vi "Demo_Ita.vi"() -> ()   [LabVIEW 2019]
uses:
  ByteQXAPIBase/ByteQXAPIBase.lvclass
  ByteQXAPIBase/FetchCalibration/Converted_Slug_Cluster.ctl
  ByteQXAPIBase/CalibrationMeasurements/CalibMeasure.ctl
  6d3d0a70-a223-4ddd-b0d3-7207305fe689.vi
  85eea304-0067-4311-882a-d02f57de18c2.vi
panel:
  out "Valore misurato":string
  out "Valore di riferimento":string
  in  "Start":bool
  in  "Send":bool
  out "Infobox":string
  out "Strumenti da calibrare":i32(listbox)
  in  "Exit":bool=TRUE
  in  "Calibrate":bool
  in  "error out":errorcluster
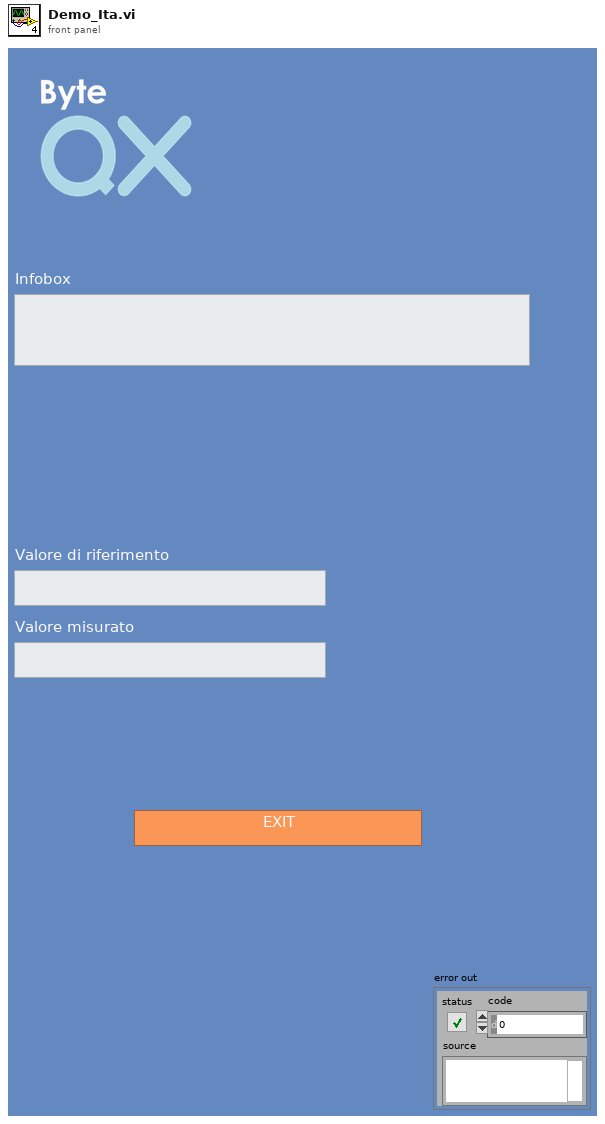
[diagram p1: front panel]
types:
  T1 = cluster{"nome":string, cluster{"Measurement_Id":i32, "Passed?":bool}[]}[]
  T2 = typedef "ByteQXWebAPI.lvlib/ByteQXAPIBase.lvclass/CalibMeasure.ctl" = cluster{"controls":cluster{"id":u16, "descrizione":string, "numero_misure_necessarie":u16, "riferimento_obiettivo":dbl, "mpe_max":dbl, "mpe_min":dbl, "deviazione_standard":dbl, "incertezza":dbl, "numero_misure_effettuate":u32, "temperatura_c":dbl, "umidita":dbl, "strumento_riferimento":cluster{"id":u16, "nome":string}[]}[]}
  T3 = typedef "ByteQXWebAPI.lvlib/ByteQXAPIBase.lvclass/Converted_Slug_Cluster.ctl" = cluster{"id":u32, "instrument":string, "name":string, "date":timestamp}
  T4 = cluster{"ByteQXAPIBase in":refnum<class "ByteQXAPIBase.lvclass">, "Expired_Instruments":T3[], "Calibrations":T2, "Strumenti_calibrati":cluster{"nome":string, cluster{"Measurement_Id":i32, "Passed?":bool}[]}[], "Instr_index":i32, "Calib_index":i32, "Instruments_Slug":string[], "ID_failed":u32, "Measure_Index":u32}
  T5 = cluster{"id":u16, "descrizione":string, "numero_misure_necessarie":u16, "riferimento_obiettivo":dbl, "mpe_max":dbl, "mpe_min":dbl, "deviazione_standard":dbl, "incertezza":dbl, "numero_misure_effettuate":u32, "temperatura_c":dbl, "umidita":dbl, "strumento_riferimento":cluster{"id":u16, "nome":string}[]}[]
  T6 = cluster{"id":u16, "descrizione":string, "numero_misure_necessarie":u16, "riferimento_obiettivo":dbl, "mpe_max":dbl, "mpe_min":dbl, "deviazione_standard":dbl, "incertezza":dbl, "numero_misure_effettuate":u32, "temperatura_c":dbl, "umidita":dbl, "strumento_riferimento":cluster{"id":u16, "nome":string}[]}
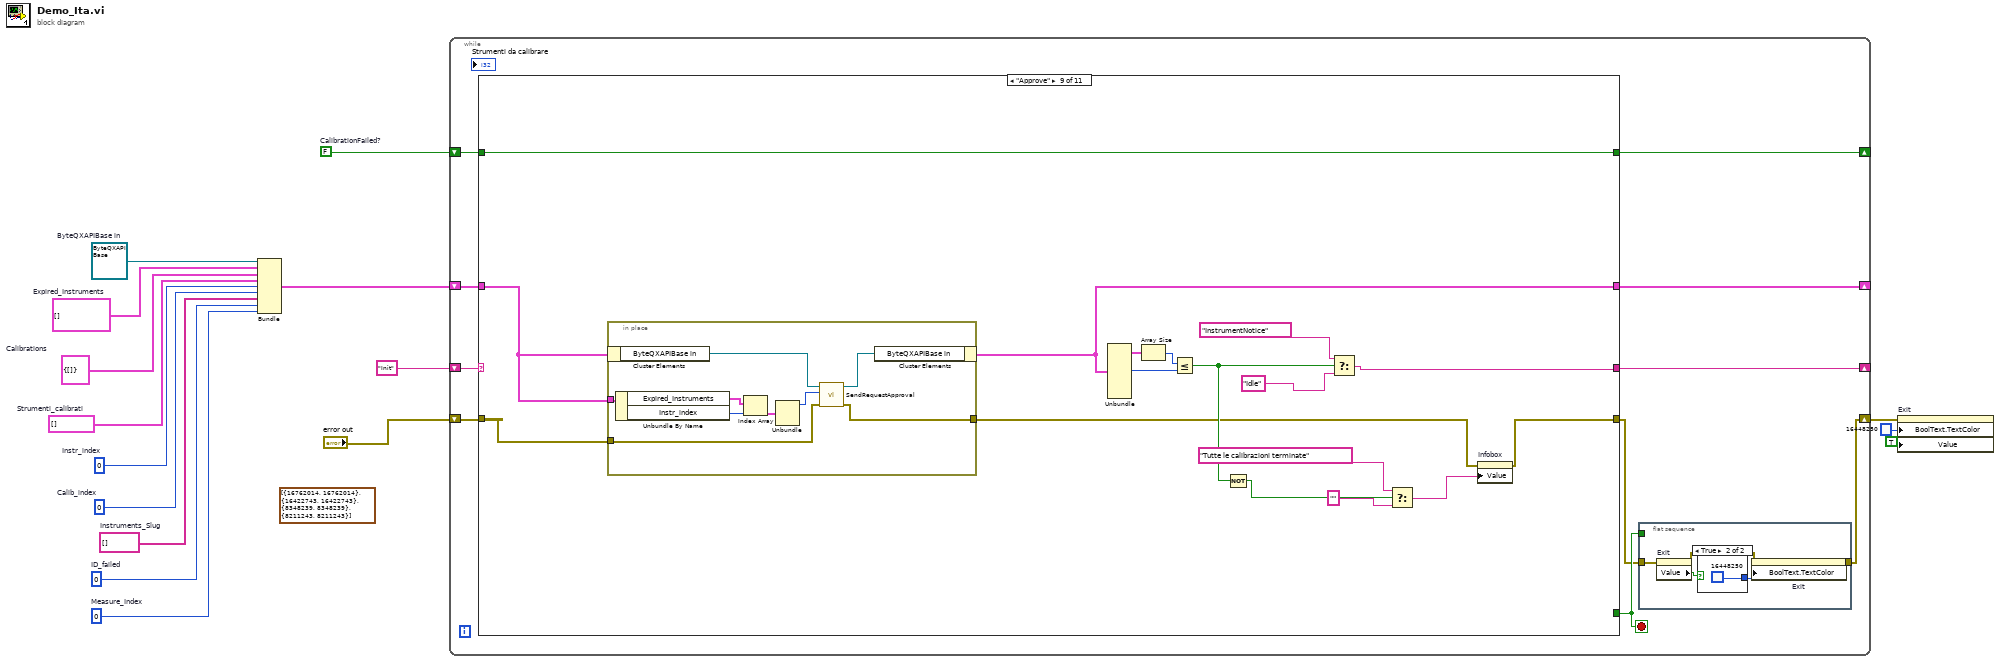
[diagram p0: block diagram]
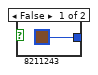
[diagram p2: hidden frame]
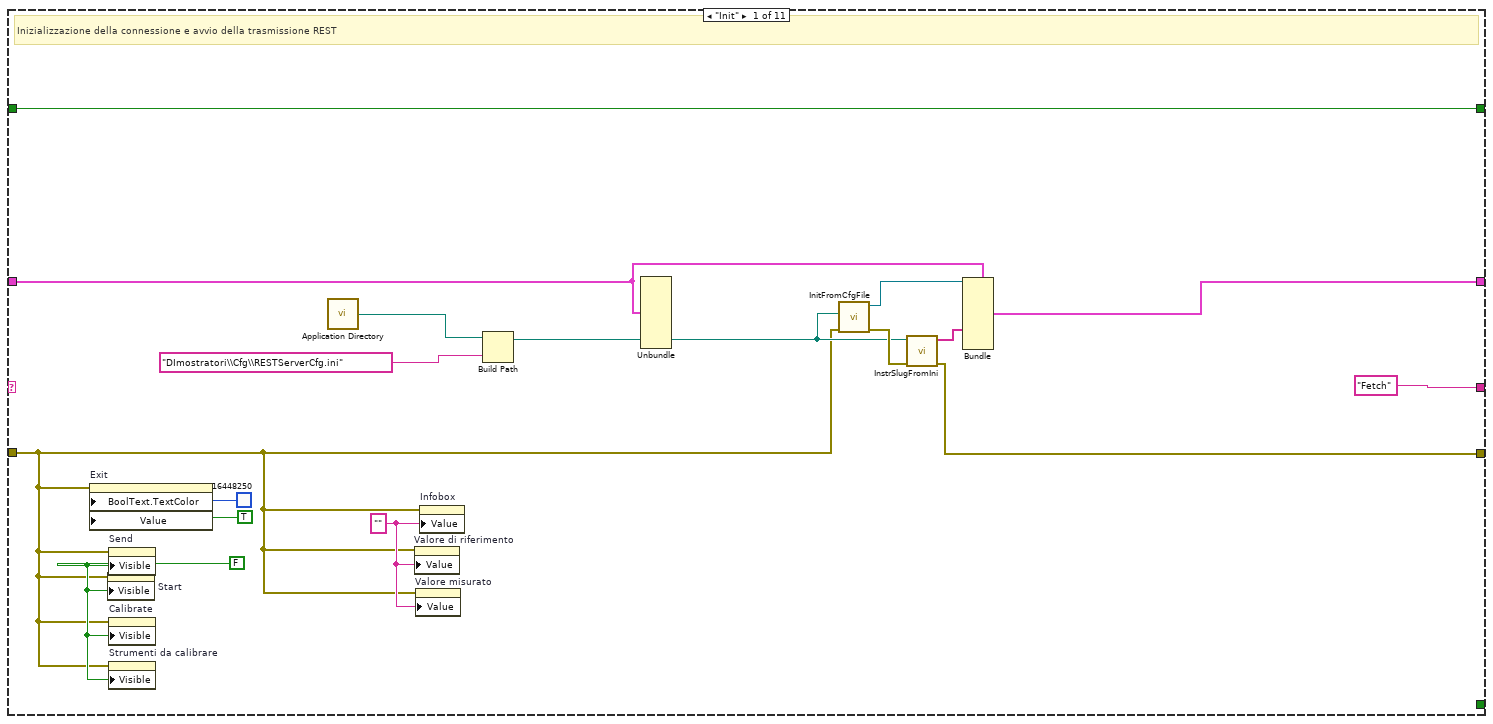
[diagram p3: hidden frame]
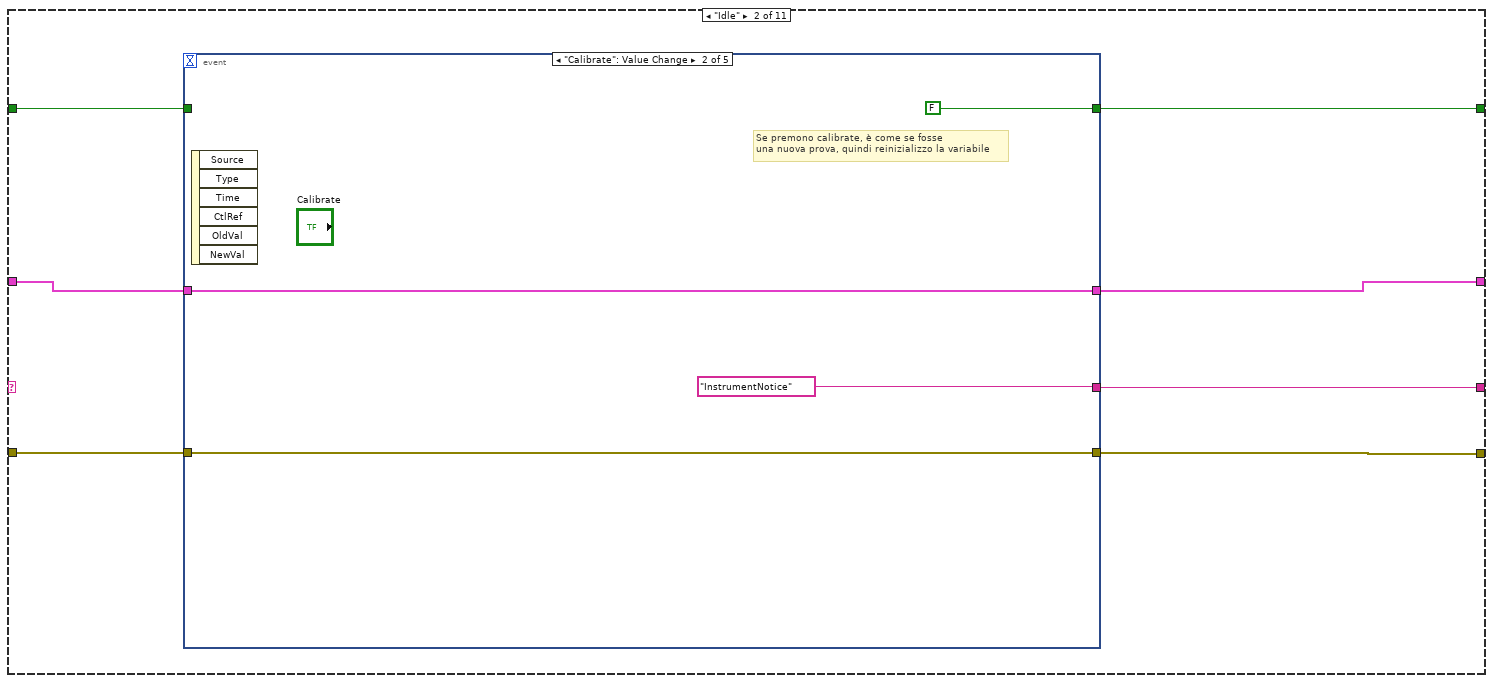
[diagram p4: hidden frame]
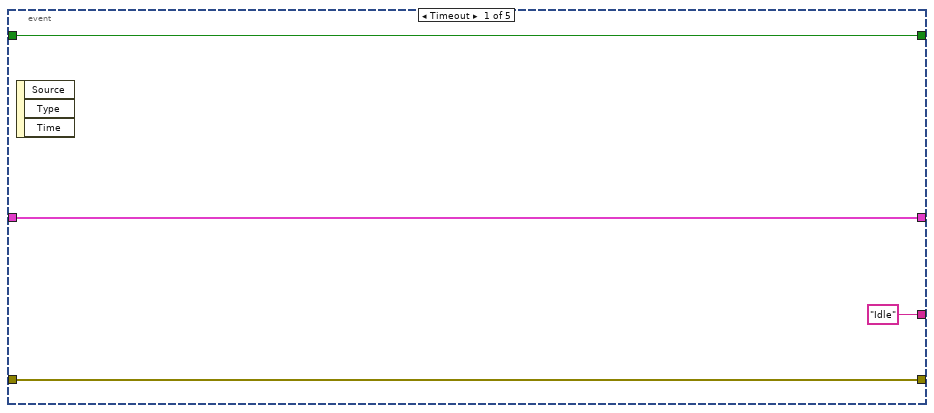
[diagram p5: hidden frame]
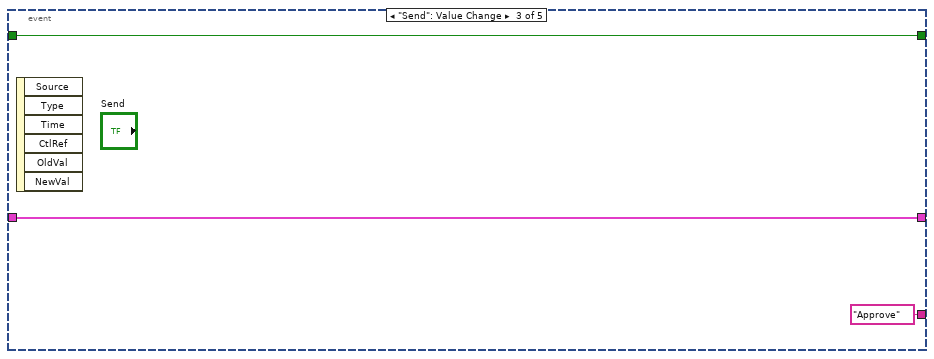
[diagram p6: hidden frame]
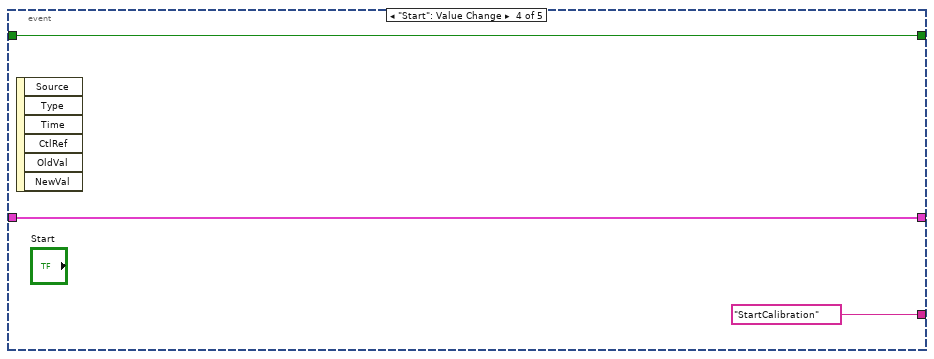
[diagram p7: hidden frame]
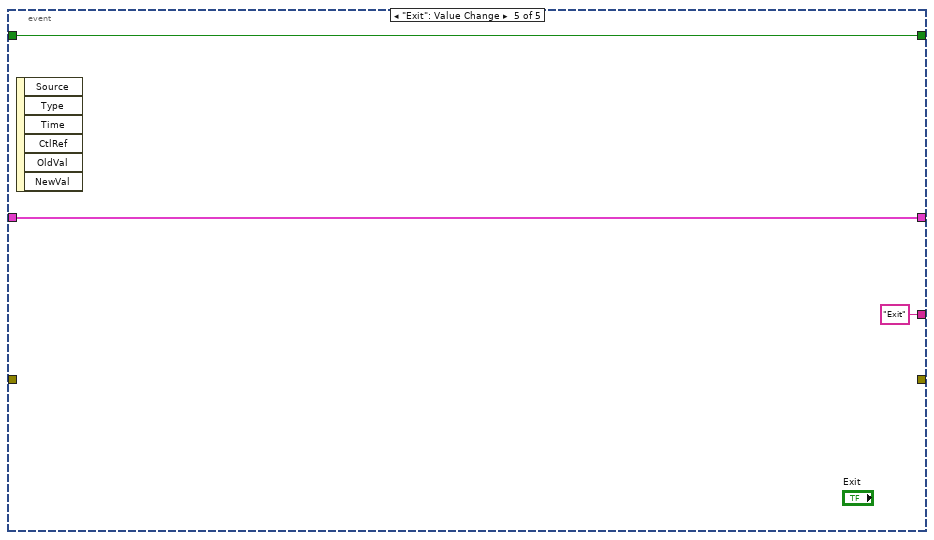
[diagram p8: hidden frame]
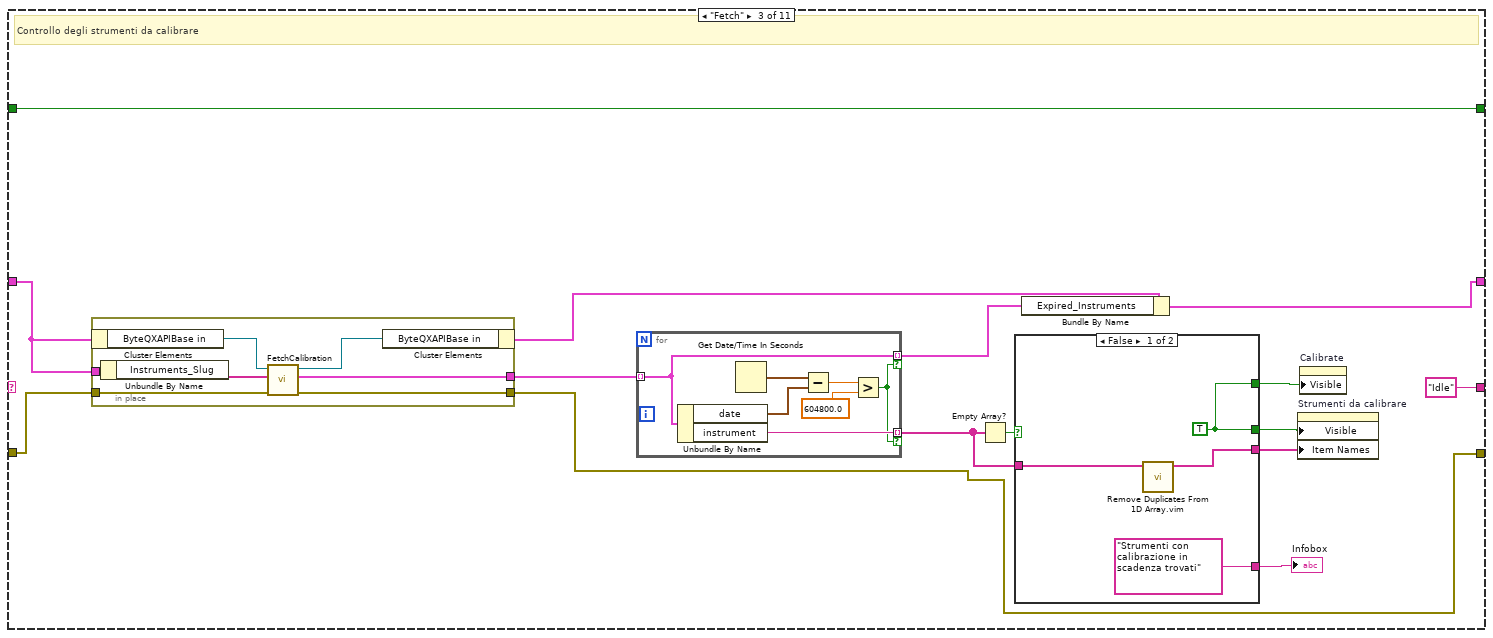
[diagram p9: hidden frame]
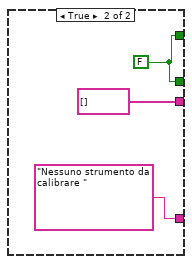
[diagram p10: hidden frame]
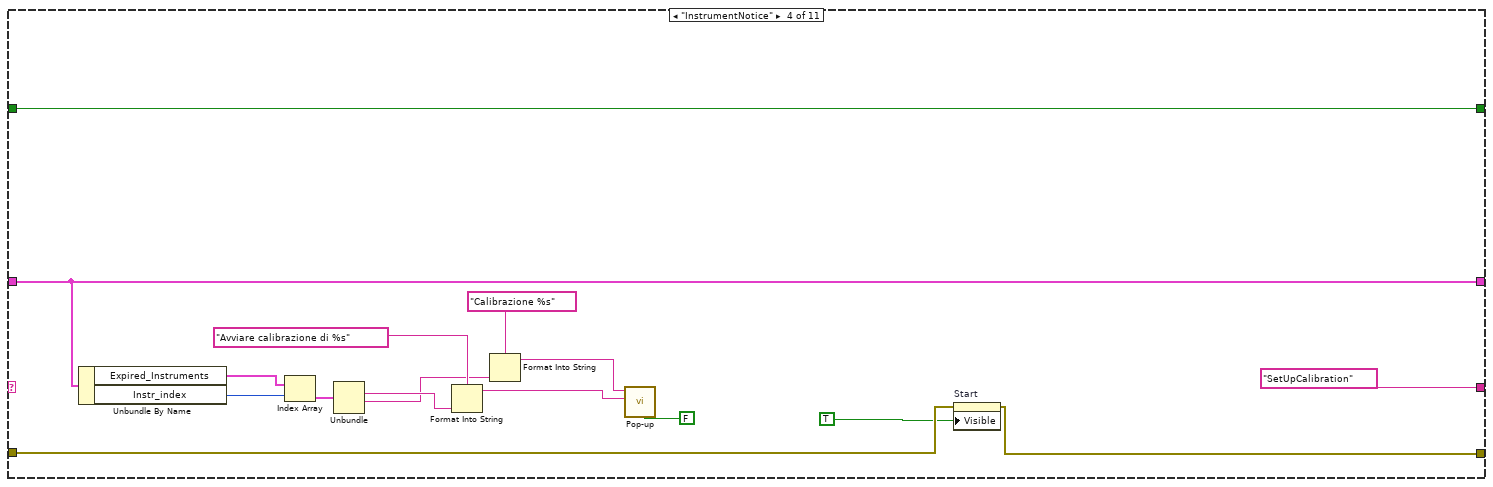
[diagram p11: hidden frame]
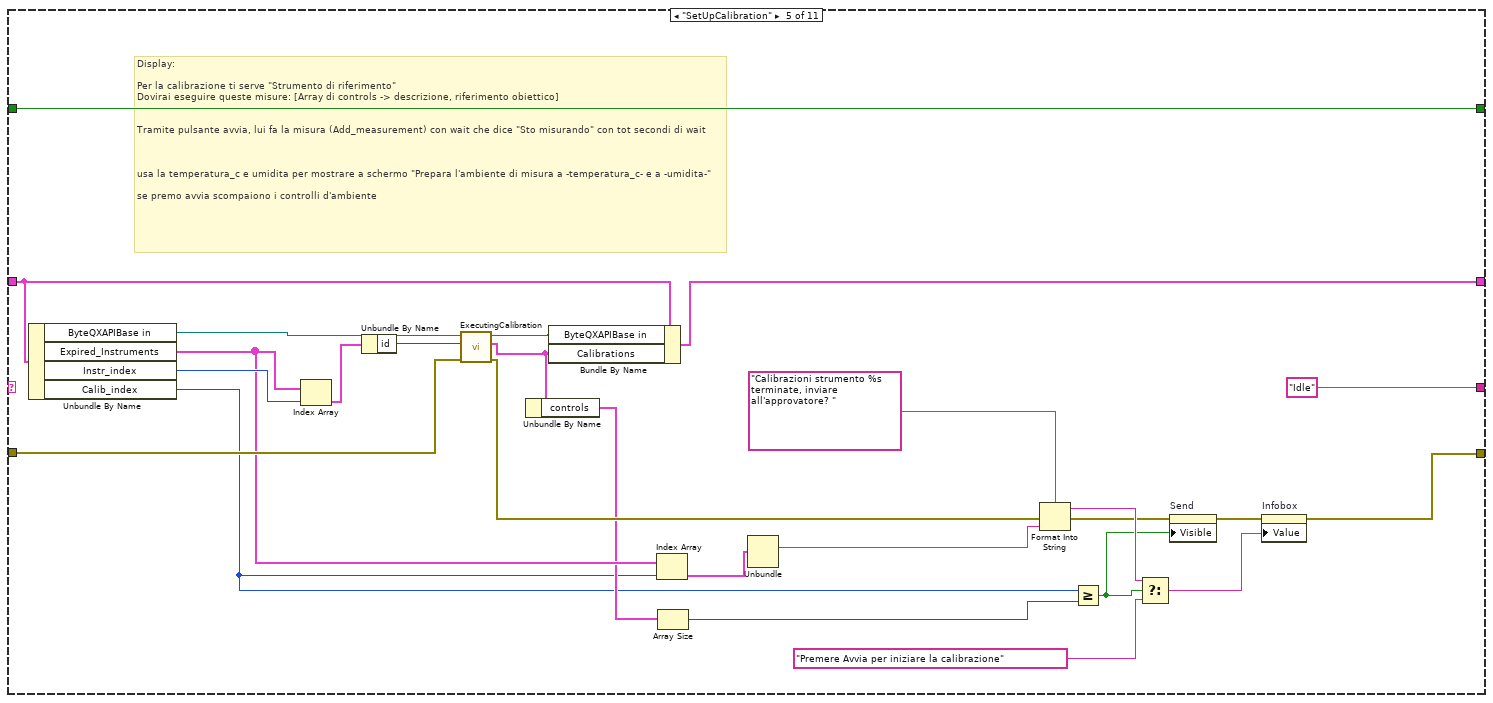
[diagram p12: hidden frame]
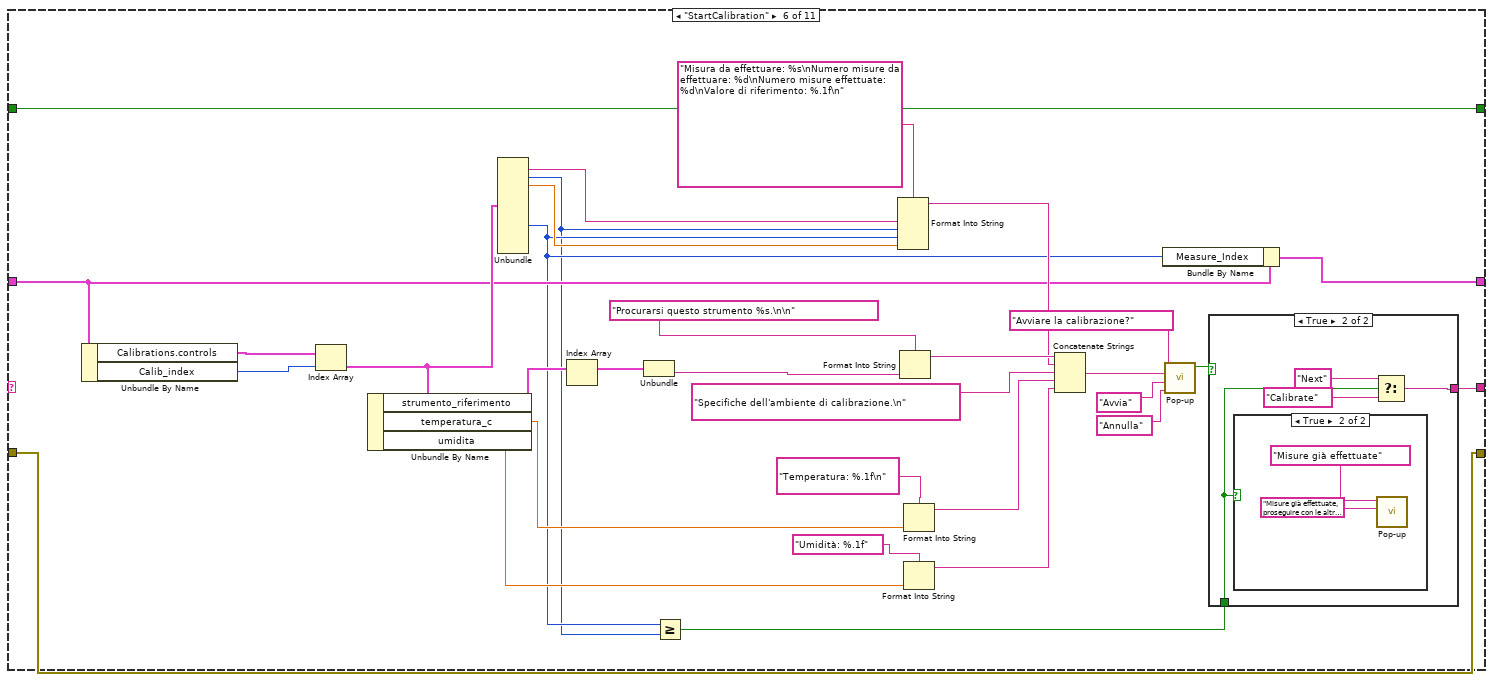
[diagram p13: hidden frame]
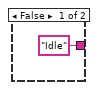
[diagram p14: hidden frame]
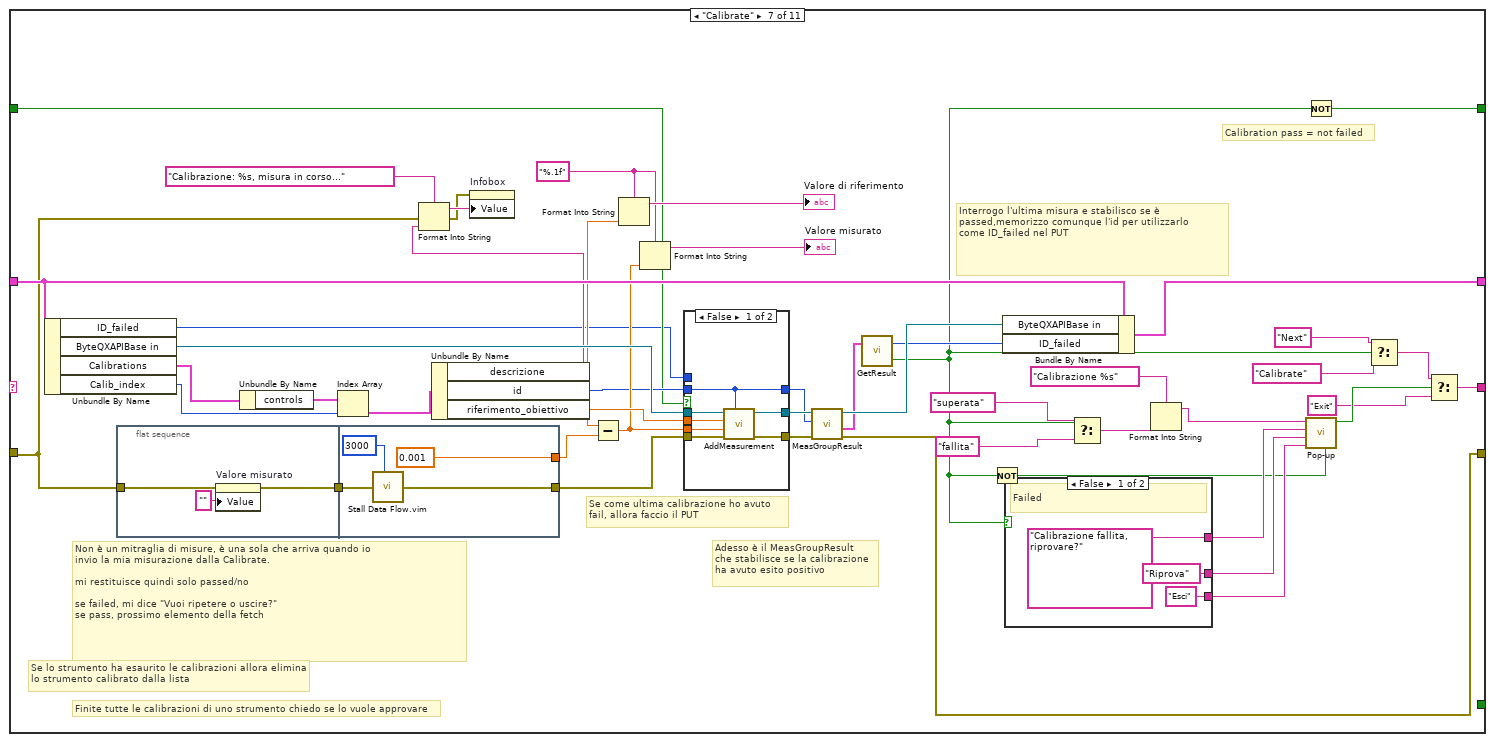
[diagram p16: hidden frame]
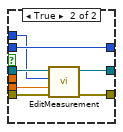
[diagram p17: hidden frame]
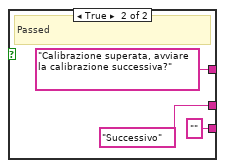
[diagram p18: hidden frame]
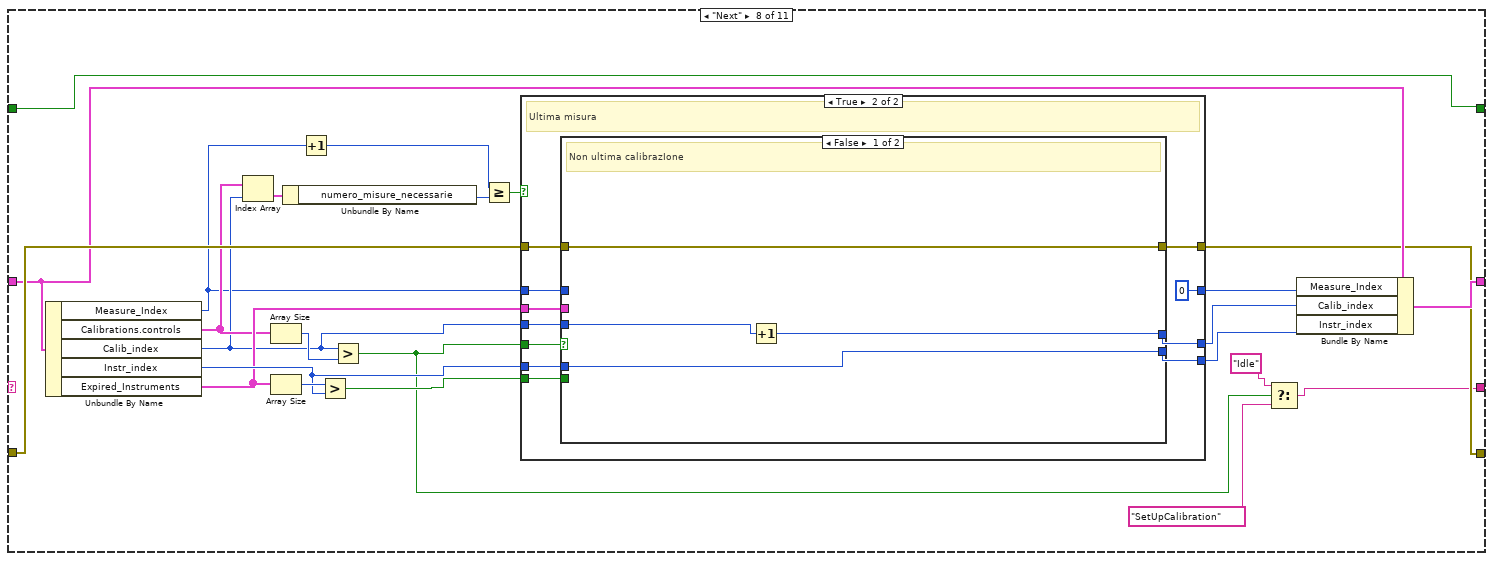
[diagram p19: hidden frame]
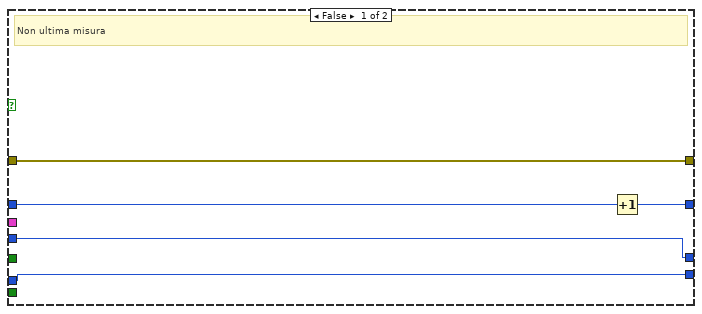
[diagram p20: hidden frame]
diagram:
  w1 = u32 0  # Measure_Index
  w2 = u32 0  # ID_failed
  w3 = FALSE  # CalibrationFailed?
  w4 = string[] []  # Instruments_Slug
  w8 = 0  # Calib_index
  w9 = 0  # Instr_index
  w10 = T1 []  # Strumenti_calibrati
  w11 = T2 {"controls"=[]}  # Calibrations
  (unwired) cluster{u32, u32}[] [{16762014, 16762014}, {16422743, 16422743}, {8348239, 8348239}, {8211243, 8211243}] ("Colors [4]")
  w12 = T3[] []  # Expired_Instruments
  w15 = refnum<class "ByteQXAPIBase.lvclass"> refnum  # ByteQXAPIBase in
  n1 = Bundle("ByteQXAPIBase in"=w15, "Expired_Instruments"=w12, "Calibrations"=w11, "Strumenti_calibrati"=w10, "Instr_index"=w9, "Calib_index"=w8, "Instruments_Slug"=w4, "ID_failed"=w2, "Measure_Index"=w1) -> (w14:T4)  [unwired: 1 in]
  n2 = while {
    shift-right: [w23] -> _
    shift-left: w14 -> [w25]
    shift-right: [w19] -> w7
    shift-left: "error out" -> [w24]
    shift-right: [w22] -> _
    shift-left: "Init" -> [w26]
    shift-right: [w17] -> _
    shift-left: w3 -> [w18]
    stop <- w21 stop-if-true
    n3 = case shown="\"Approve\"" w26 {
      tunnel: w25 -> [w49 w53 w75 w125 w151 w156 w237 w281 w338 w351 w355]
      tunnel: w24 -> [w37 w55 w88 w113 w147 w175 w206 w282 w337 w352 w356]
      tunnel: [w40 w56 w76 w112 w143 w175 w202 w280 w323 w352 w356] -> w20
      tunnel: [w48 w54 w77 w125 w149 w155 w207 w287 w336 w351 w355] -> w23
      tunnel: [_ _ _ _ _ _ _ _ _ TRUE _] -> w21
      tunnel: ["Fetch" w52 "Idle" ("t") "SetUpCalibration" ("t") "Idle" ("t") w169 w213 w275 w330 "" ("t") "Exit" ("t")] -> w22
      tunnel: w18 -> [w36 w51 w74 w110 w129 w163 w197 w273 w322 w348 w353]
      tunnel: [w36 w50 w74 w110 w129 w163 w196 w273 w322 w348 w353] -> w17
      frame "Init" {
        w44 = "" ("Infobox")
        w43 = FALSE
        # "Inizializzazione della connessione e avvio della trasmissione REST"
        n4 = property on="Exit" class="Bool (strict)"(error in=w37, "BoolText.TextColor"=u32 16448250, "Value"=TRUE ("Exit")) -> ()  [unwired: 1 in, 2 out]
        n5 = property on="Start" class="Bool"(error in=w37, "Visible"=w43) -> ()  [unwired: 1 in, 2 out]
        n6 = property on="Send" class="Bool"(error in=w37, "Visible"=w43) -> ()  [unwired: 1 in, 2 out]
        n7 = property on="Calibrate" class="Bool"(error in=w37, "Visible"=w43) -> ()  [unwired: 1 in, 2 out]
        n8 = property on="Strumenti da calibrare" class="LstBox (strict)"(error in=w37, "Visible"=w43) -> ()  [unwired: 1 in, 2 out]
        n9 = call <vilib>:"Application Directory.vi"() -> ("Application Directory"=w35:path)
        n10 = property on="Valore di riferimento" class="Str"(error in=w37, "Value"=w44) -> ()  [unwired: 1 in, 2 out]
        n11 = property on="Valore misurato" class="Str"(error in=w37, "Value"=w44) -> ()  [unwired: 1 in, 2 out]
        n12 = property on="Infobox" class="Str"(error in=w37, "Value"=w44) -> ()  [unwired: 1 in, 2 out]
        n13 = Build Path(base path=w35, name or relative path="DImostratori\\Cfg\\RESTServerCfg.ini") -> (appended path=w39:path)
        n14 = Unbundle(w49) -> ()  [unwired: 9 out]
        n15 = call "InitFromCfgFile.vi"("error in (no error)"=w37, "configuration file path"=w39) -> ("error out"=w41:errorcluster, "ByteQXAPIBase out"=w34:refnum<class "ByteQXAPIBase.lvclass">)  [unwired: 8 in]
        n16 = call "InstrSlugFromIni.vi"("error in (no error)"=w41, "configuration file path"=w39) -> ("error out"=w40:errorcluster, "Array"=w38:string[])  [unwired: 8 in]
        n17 = Bundle(cluster=w49, "ByteQXAPIBase in"=w34, "Instruments_Slug"=w38) -> (w48:T4)  [unwired: 7 in]
      }
      frame "Idle" {
        n18 = event shown="[1] \"Calibrate\": Value Change" {
          selector: _ -> [_ _ _ _ _]
          dyn-events: _ -> [_ _ _ _ _]
          timeout: _ -> [_ _ _ _ _]
          tunnel: [w60 w62 _ _ _] -> w56
          tunnel: w55 -> [w60 w62 _ _ _]
          tunnel: [w59 w64 w67 w70 w73] -> w54
          tunnel: w53 -> [w59 w64 w67 w70 w73]
          tunnel: ["Idle" ("t") "InstrumentNotice" "Approve" ("t") "StartCalibration" ("t") "Exit" ("t")] -> w52
          tunnel: w51 -> [w57 _ w65 w68 w71]
          tunnel: [w57 FALSE ("CalibrationFailed?") w65 w68 w71] -> w50
          event Timeout {
            n19 = event-data() -> ()  [unwired: 1 in, 3 out]
          }
          event "Calibrate": Value Change {
            # "Se premono calibrate, è come se fosse\nuna nuova prova, quindi reinizializzo la variabile"
            n20 = event-data() -> ()  [unwired: 1 in, 6 out]
          }
          event "Send": Value Change {
            n21 = event-data() -> ()  [unwired: 1 in, 6 out]
          }
          event "Start": Value Change {
            n22 = event-data() -> ()  [unwired: 1 in, 6 out]
          }
          event "Exit": Value Change {
            n23 = event-data() -> ()  [unwired: 1 in, 6 out]
          }
        }
      }
      frame "Fetch" {
        # "Controllo degli strumenti da calibrare"
        n24 = in-place {
          in-place-border: w88 -> [w94]
          in-place-border: [w93] -> w76
          in-place-border: [w92] -> w80
          in-place-border: w75 -> [w90]
          n25 = in-place-cluster #1(w75) -> ("ByteQXAPIBase in"=w91:refnum<class "ByteQXAPIBase.lvclass">)
          n26 = Unbundle By Name(w90) -> ("Instruments_Slug"=w89:string[])
          n27 = call-dynamic "FetchCalibration.vi"("error in (no error)"=w94, "instruments"=w89, "ByteQXAPIBase in"=w91) -> ("error out"=w93:errorcluster, "instruments"=w92:T3[], "ByteQXAPIBase out"=w95:refnum<class "ByteQXAPIBase.lvclass">)  [unwired: 6 in]
          n28 = in-place-cluster #1("ByteQXAPIBase in"=w95) -> (w87:T4)
        }
        n29 = for {
          tunnel: w80 -> [w98] mode=indexing
          tunnel: [w98] -> w79 mode=indexing if=w96
          tunnel: [w97] -> w85 mode=indexing if=w96
          n30 = Unbundle By Name(w98) -> ("date"=w99:timestamp, "instrument"=w97:string)
          n31 = Get Date/Time In Seconds() -> (seconds since 1Jan1904=w101:timestamp)
          n32 = Subtract(x=w101, y=w99) -> (x-y=w102:dbl)
          n33 = Greater?(x=w102, y=604800.0) -> (0:w96:bool)
        }
        n34 = Empty Array?(array=w85) -> (empty?=w86:bool)
        n35 = case shown="False" w86 {
          tunnel: w85 -> [w105 _]
          tunnel: [w103 w107] -> w84
          tunnel: ["Strumenti con calibrazione in scadenza trovati" ("Infobox") "Nessuno strumento da calibrare " ("Infobox")] -> w83
          tunnel: [w104 string[] []] -> w82
          tunnel: [w103 w107] -> w78
          frame False {
            w103 = TRUE ("Visible")
            n36 = call "Remove Duplicates From 1D Array.vim"("array"=w105) -> ("array with duplicates removed"=w104:string[])  [unwired: 10 in]
          }
          frame True {
            w107 = FALSE ("Visible")
          }
        }
        "Infobox" <- w83
        n37 = Bundle By Name(cluster=w87, "Expired_Instruments"=w79) -> (w77:T4)
        n38 = property on="Strumenti da calibrare" class="LstBox (strict)"("Visible"=w84, "Item Names"=w82) -> ()  [unwired: 2 in, 2 out]
        n39 = property on="Calibrate" class="Bool"("Visible"=w78) -> ()  [unwired: 2 in, 2 out]
      }
      frame "InstrumentNotice" {
        n40 = Unbundle By Name(w125) -> ("Expired_Instruments"=w124:T3[], "Instr_index"=w123:i32)
        n41 = Index Array(array=w124, index=w123) -> (element=w122:T3)
        n42 = Unbundle(w122) -> ("instrument"=w120:string, "name"=w118:string)  [unwired: 2 out]
        n43 = Format Into String(format string="Avviare calibrazione di %s" ("Title"), w120) -> (resulting string=w119:string)  [unwired: 2 in, 1 out]
        n44 = Format Into String(format string="Calibrazione %s", w118) -> (resulting string=w116:string)  [unwired: 2 in, 1 out]
        n45 = call "Pop-up.vi"("Two_btn"=FALSE, "Text"=w119, "Title"=w116) -> ()  [unwired: 8 in, 1 out]
        n46 = property on="Start" class="Bool"(error in=w113, "Visible"=TRUE) -> (error out=w112:errorcluster)  [unwired: 1 in, 1 out]
      }
      frame "SetUpCalibration" {
        # "Display: \n\nPer la calibrazione ti serve \"Strumento di riferimento\"\nDovirai eseguire queste misure: [Array di controls -> descrizione, riferimento obiettico] \n\n\nTramite pulsante avvia, lui fa la misura (Add_measurement) con wait che dice \"Sto misurando\" con tot secondi di wait\n\n\n\nusa la temperatura_c e umidita per mostrare a schermo \"Prepara l'ambiente di misura a -temperatura_c- e a -umidita-\"\n\nse premo avvia scompaiono i controlli d'ambiente"
        n47 = Unbundle By Name(w151) -> ("ByteQXAPIBase in"=w150:refnum<class "ByteQXAPIBase.lvclass">, "Expired_Instruments"=w139:T3[], "Instr_index"=w144:i32, "Calib_index"=w127:i32)
        n48 = Index Array(array=w139, index=w144) -> (element=w145:T3)
        n49 = Unbundle By Name(w145) -> ("id"=w126:u32)
        n50 = call-dynamic "ExecutingCalibration.vi"("error in (no error)"=w147, "calibration_id"=w126, "ByteQXAPIBase in"=w150) -> ("error out"=w133:errorcluster, "calibration data"=w128:T2, "ByteQXAPIBase out"=w148:refnum<class "ByteQXAPIBase.lvclass">)  [unwired: 6 in]
        n51 = Unbundle By Name(w128) -> ("controls"=w130:T5)
        n52 = Bundle By Name(cluster=w151, "ByteQXAPIBase in"=w148, "Calibrations"=w128) -> (w149:T4)
        n53 = Index Array(array=w139, index=w127) -> (element=w140:T3)
        n54 = Array Size(array=w130) -> (size(s)=w137:i32)
        n55 = Unbundle(w140) -> ("instrument"=w138:string)  [unwired: 3 out]
        n56 = Format Into String(format string="Calibrazioni strumento %s terminate, inviare all'approvatore? ", error in=w133, w138) -> (resulting string=w142:string, error out=w132:errorcluster)  [unwired: 1 in]
        n57 = Greater Or Equal?(x=w127, y=w137) -> (x >= y?=w134:bool)
        n58 = Select(t=w142, s=w134, f="Premere Avvia per iniziare la calibrazione" ("Infobox")) -> (s? t:f=w135:string)
        n59 = property on="Send" class="Bool"(error in=w132, "Visible"=w134) -> (error out=w131:errorcluster)  [unwired: 1 in, 1 out]
        n60 = property on="Infobox" class="Str"(error in=w131, "Value"=w135) -> (error out=w143:errorcluster)  [unwired: 1 in, 1 out]
      }
      frame "StartCalibration" {
        n61 = Unbundle By Name(w156) -> ("Calibrations.controls"=w167:T5, "Calib_index"=w168:i32)
        n62 = Index Array(array=w167, index=w168) -> (element=w162:T6)
        n63 = Unbundle By Name(w162) -> ("strumento_riferimento"=w159:cluster{"id":u16, "nome":string}[], "temperatura_c"=w161:dbl, "umidita"=w160:dbl)
        n64 = Unbundle(w162) -> ("descrizione"=w165:string, "numero_misure_necessarie"=w153:u16, "riferimento_obiettivo"=w157:dbl, "numero_misure_effettuate"=w154:u32)  [unwired: 8 out]
        n65 = Index Array(array=w159) -> (element=w158:cluster{"id":u16, "nome":string})  [unwired: 1 in]
        n66 = Unbundle(w158) -> ("nome"=w177:string)  [unwired: 1 out]
        n67 = Greater Or Equal?(x=w154, y=w153) -> (x >= y?=w152:bool)
        n68 = Format Into String(format string="Misura da effettuare: %s\nNumero misure da effettuare: %d\nNumero misure effettuate: %d\nValore di riferimento: %.1f\n", w165, w153, w154, w157) -> (resulting string=w166:string)  [unwired: 2 in, 1 out]
        n69 = Format Into String(format string="Procurarsi questo strumento %s.\n\n", w177) -> (resulting string=w183:string)  [unwired: 2 in, 1 out]
        n70 = Format Into String(format string="Temperatura: %.1f\n", w161) -> (resulting string=w174:string)  [unwired: 2 in, 1 out]
        n71 = Format Into String(format string="Umidità: %.1f", w160) -> (resulting string=w172:string)  [unwired: 2 in, 1 out]
        n72 = Concatenate Strings(w183, w166, "Specifiche dell'ambiente di calibrazione.\n" ("string"), w174, w172) -> (w178:string)
        n73 = Bundle By Name(cluster=w156, "Measure_Index"=w154) -> (w155:T4)
        n74 = call "Pop-up.vi"("CancelText"="Annulla", "OkText"="Avvia", "Text"=w178, "Title"="Avviare la calibrazione?") -> ("Btn-OK Out"=w170:bool)  [unwired: 7 in]
        n75 = case shown="True" w170 {
          tunnel: ["Idle" w186] -> w169
          tunnel: w152 -> [_ w185]
          frame False {
          }
          frame True {
            n76 = case shown="True" w185 {
              frame False {
              }
              frame True {
                n77 = call "Pop-up.vi"("Text"="Misure già effettuate, proseguire con le altre tarature" ("Title"), "Title"="Misure già effettuate") -> ()  [unwired: 9 in, 1 out]
              }
            }
            n78 = Select(t="Next", s=w185, f="Calibrate") -> (s? t:f=w186:string)
          }
        }
      }
      frame "Calibrate" {
        w226 = "%.1f" ("format string")
        # "Interrogo l'ultima misura e stabilisco se è passed,memorizzo comunque l'id per utilizzarlo\ncome ID_failed nel PUT"
        # "Calibration pass = not failed"
        # "Se come ultima calibrazione ho avuto\nfail, allora faccio il PUT"
        # "Adesso è il MeasGroupResult\nche stabilisce se la calibrazione\nha avuto esito positivo"
        # "Finite tutte le calibrazioni di uno strumento chiedo se lo vuole approvare"
        # "Se lo strumento ha esaurito le calibrazioni allora elimina\nlo strumento calibrato dalla lista"
        # "Non è un mitraglia di misure, è una sola che arriva quando io\ninvio la mia misurazione dalla Calibrate.\n\nmi restituisce quindi solo passed/no \n\nse failed, mi dice \"Vuoi ripetere o uscire?\"\nse pass, prossimo elemento della fetch"
        n79 = Unbundle By Name(w237) -> ("ID_failed"=w191:u32, "ByteQXAPIBase in"=w236:refnum<class "ByteQXAPIBase.lvclass">, "Calibrations"=w235:T2, "Calib_index"=w229:i32)
        n80 = flat-sequence {
          tunnel: w206 -> [w253]
          tunnel: [w254] -> w204
          tunnel: [0.001 ("number: 0 to 1")] -> w224
          tunnel: [w256] -> w205
          tunnel: w204 -> [w257]
          frame #0 {
            n81 = property on="Valore misurato" class="Str"(error in=w253, "Value"="" ("Valore misurato")) -> (error out=w254:errorcluster)  [unwired: 1 in, 1 out]
          }
          frame #1 {
            n82 = call "Stall Data Flow.vim"("value in"=w257, "milliseconds to wait"=u32 3000) -> ("value out"=w256:errorcluster)  [unwired: 1 out]
          }
        }
        n83 = Unbundle By Name(w235) -> ("controls"=w230:T5)
        n84 = Index Array(array=w230, index=w229) -> (element=w231:T6)
        n85 = Unbundle By Name(w231) -> ("descrizione"=w195:string, "id"=w201:u16, "riferimento_obiettivo"=w228:dbl)
        n86 = Format Into String(format string="Calibrazione: %s, misura in corso...", error in=w206, w195) -> (resulting string=w234:string, error out=w233:errorcluster)  [unwired: 1 in]
        n87 = property on="Infobox" class="Str"(error in=w233, "Value"=w234) -> ()  [unwired: 1 in, 2 out]
        n88 = Subtract(x=w228, y=w224) -> (x-y=w208:dbl)
        n89 = Format Into String(format string=w226, w228) -> (resulting string=→"Valore di riferimento":string)  [unwired: 2 in, 1 out]
        n90 = Format Into String(format string=w226, w208) -> (resulting string=→"Valore misurato":string)  [unwired: 2 in, 1 out]
        n91 = case shown="False" w197 {
          tunnel: w236 -> [w244 w251]
          tunnel: w228 -> [w243 _]
          tunnel: w208 -> [w242 w249]
          tunnel: w205 -> [w241 w250]
          tunnel: [w240 w247] -> w203
          tunnel: w201 -> [w238 w246]
          tunnel: [w239 w248] -> w200
          tunnel: [w238 w246] -> w198
          tunnel: w191 -> [_ w245]
          frame False {
            n92 = call-dynamic "AddMeasurement.vi"("measurement-group-id"=w238, "error in (no error)"=w241, "instrument measure"=w242, "reference measure"=w243, "ByteQXAPIBase in"=w244) -> ("error out"=w240:errorcluster, "ByteQXAPIBase out"=w239:refnum<class "ByteQXAPIBase.lvclass">)  [unwired: 4 in, 1 out]
          }
          frame True {
            n93 = call-dynamic "EditMeasurement.vi"("error in (no error)"=w250, "instrument measure"=w249, "measurement-id"=w245, "ByteQXAPIBase in"=w251) -> ("error out"=w247:errorcluster, "ByteQXAPIBase out"=w248:refnum<class "ByteQXAPIBase.lvclass">)  [unwired: 5 in, 1 out]
          }
        }
        n94 = call-dynamic "MeasGroupResult.vi"("error in (no error)"=w203, "measurement_group_id"=w198, "ByteQXAPIBase in"=w200) -> ("error out"=w202:errorcluster, "measurements"=w194:cluster{"id":u32, "passed":bool}[], "ByteQXAPIBase out"=w199:refnum<class "ByteQXAPIBase.lvclass">)  [unwired: 5 in, 1 out]
        n95 = call "GetResult.vi"("measurements"=w194) -> ("passed"=w192:bool, "id"=w193:u32)  [unwired: 1 in]
        n96 = Not(x=w192) -> (.not. x?=w212:bool)
        n97 = Bundle By Name(cluster=w237, "ByteQXAPIBase in"=w199, "ID_failed"=w193) -> (w207:T4)
        n98 = case shown="False" w192 {
          tunnel: ["Riprova" "Successivo"] -> w218
          tunnel: ["Esci" ""] -> w217
          tunnel: ["Calibrazione fallita, riprovare?" ("Text") "Calibrazione superata, avviare la calibrazione successiva?" ("Text")] -> w216
          frame False {
            # "Failed"
          }
          frame True {
            # "Passed"
          }
        }
        n99 = Select(t="superata", s=w192, f="fallita") -> (s? t:f=w222:string)
        n100 = Format Into String(format string="Calibrazione %s", w222) -> (resulting string=w219:string)  [unwired: 2 in, 1 out]
        n101 = Not(x=w192) -> (.not. x?=w196:bool)
        n102 = call "Pop-up.vi"("Two_btn"=w212, "CancelText"=w217, "OkText"=w218, "Text"=w216, "Title"=w219) -> ("Btn-OK Out"=w215:bool)  [unwired: 6 in]
        n103 = Select(t="Next", s=w192, f="Calibrate") -> (s? t:f=w210:string)
        n104 = Select(t=w210, s=w215, f="Exit") -> (s? t:f=w213:string)
      }
      frame "Next" {
        n105 = Unbundle By Name(w281) -> ("Measure_Index"=w267:u32, "Calibrations.controls"=w272:T5, "Calib_index"=w271:i32, "Instr_index"=w283:i32, "Expired_Instruments"=w279:T3[])
        n106 = Index Array(array=w272, index=w271) -> (element=w270:T6)
        n107 = Array Size(array=w272) -> (size(s)=w288:i32)
        n108 = Array Size(array=w279) -> (size(s)=w285:i32)
        n109 = Unbundle By Name(w270) -> ("numero_misure_necessarie"=w269:u16)
        n110 = Increment(x=w267) -> (x+1=w265:u32)
        n111 = Greater?(x=w285, y=w283) -> (0:w278:bool)
        n112 = Greater?(x=w271, y=w288) -> (0:w274:bool)
        n113 = Greater Or Equal?(x=w265, y=w269) -> (x >= y?=w268:bool)
        n114 = case shown="True" w268 {
          tunnel: [w293 w304] -> w286
          tunnel: [w292 w303] -> w284
          tunnel: w271 -> [w293 w302]
          tunnel: w283 -> [w292 w301]
          tunnel: w282 -> [w289 w300]
          tunnel: [w289 w299] -> w280
          tunnel: w279 -> [_ w298]
          tunnel: w278 -> [_ w297]
          tunnel: w274 -> [_ w296]
          tunnel: w267 -> [w291 w294]
          tunnel: [w290 u32 0] -> w266
          frame False {
            # "Non ultima misura"
            n115 = Increment(x=w291) -> (x+1=w290:u32)
          }
          frame True {
            # "Ultima misura"
            n116 = case shown="False" w296 {
              tunnel: [w307 0 ("Calib_index")] -> w304
              tunnel: w302 -> [w308 _]
              tunnel: w301 -> [w306 w314]
              tunnel: w297 -> [_ w316]
              tunnel: [w306 w313] -> w303
              tunnel: w300 -> [w305 w312]
              tunnel: [w305 w311] -> w299
              tunnel: w298 -> [_ w310]
              tunnel: w294 -> [_ w309]
              frame False {
                # "Non ultima calibrazIone"
                n117 = Increment(x=w308) -> (x+1=w307:i32)
              }
              frame True {
                # "ultima controllo"
                n118 = case shown="True" w316 {
                  tunnel: w314 -> [w319 _]
                  tunnel: [w318 0] -> w313
                  tunnel: w312 -> [w317 w320]
                  tunnel: [w317 w320] -> w311
                  tunnel: w310 -> [_ _]
                  tunnel: w309 -> [_ _]
                  frame False {
                    n119 = Increment(x=w319) -> (x+1=w318:i32)
                  }
                  frame True {
                    # "Ultimo Strumento"
                  }
                }
              }
            }
          }
        }
        n120 = Select(t="Idle", s=w274, f="SetUpCalibration") -> (s? t:f=w275:string)
        n121 = Bundle By Name(cluster=w281, "Measure_Index"=w266, "Calib_index"=w286, "Instr_index"=w284) -> (w287:T4)
      }
      frame "Approve" {
        n122 = in-place {
          in-place-border: w338 -> [w345]
          in-place-border: w337 -> [w344]
          in-place-border: [w343] -> w324
          n123 = in-place-cluster #2(w338) -> ("ByteQXAPIBase in"=w347:refnum<class "ByteQXAPIBase.lvclass">)
          n124 = Unbundle By Name(w345) -> ("Expired_Instruments"=w342:T3[], "Instr_index"=w341:i32)
          n125 = Index Array(array=w342, index=w341) -> (element=w340:T3)
          n126 = Unbundle(w340) -> ("id"=w339:u32)  [unwired: 3 out]
          n127 = call-dynamic "SendRequestApproval.vi"("error in (no error)"=w344, "calibration-id"=w339, "ByteQXAPIBase in"=w347) -> ("error out"=w343:errorcluster, "ByteQXAPIBase out"=w346:refnum<class "ByteQXAPIBase.lvclass">)  [unwired: 6 in, 1 out]
          n128 = in-place-cluster #2("ByteQXAPIBase in"=w346) -> (w336:T4)
        }
        n129 = Unbundle(w336) -> ("Expired_Instruments"=w335:T3[], "Instr_index"=w333:i32)  [unwired: 7 out]
        n130 = Array Size(array=w335) -> (size(s)=w334:i32)
        n131 = Less Or Equal?(x=w334, y=w333) -> (x <= y?=w327:bool)
        n132 = Not(x=w327) -> (.not. x?=w326:bool)
        n133 = Select(t="InstrumentNotice", s=w327, f="Idle") -> (s? t:f=w330:string)
        n134 = Select(t="Tutte le calibrazioni terminate", s=w326, f="") -> (s? t:f=w325:string)
        n135 = property on="Infobox" class="Str"(error in=w324, "Value"=w325) -> (error out=w323:errorcluster)  [unwired: 1 in, 1 out]
      }
      frame "Exit" {
        # "Uscita"
      }
      frame Default {
        # "Qua non dovrebbe entrarci"
      }
    }
    n136 = flat-sequence {
      tunnel: w21 -> [_]
      tunnel: [w29] -> w19
      tunnel: w20 -> [w28]
      frame #0 {
        n137 = property on="Exit" class="Bool (strict)"(error in=w28) -> (error out=w27:errorcluster, "Value"=w30:bool)  [unwired: 1 in, 1 out]
        n138 = case shown="True" w30 {
          tunnel: [u32 8211243 u32 16448250 ("Boolean Text.Text Colors:Text Color")] -> w31
          frame False {
          }
          frame True {
          }
        }
        n139 = property on="Exit" class="Bool (strict)"(error in=w27, "BoolText.TextColor"=w31) -> (error out=w29:errorcluster)  [unwired: 1 in, 1 out]
      }
    }
  }
  n140 = property on="Exit" class="Bool (strict)"(error in=w7, "BoolText.TextColor"=u32 16448250 ("Boolean Text.Text Colors:Text Color"), "Value"=TRUE ("Exit")) -> ()  [unwired: 1 in, 2 out]
